vi "LabVIEW Basics #1 - Arduino Blinking LED.vi"() -> ()   [LabVIEW 2019]
uses:
  <vilib>/MakerHub/LINX/Public/Peripherals/Digital/Digital Write 1 Chan.vi
  <vilib>/MakerHub/LINX/Public/Peripherals/Digital/Digital Write N Chans.vi
  <vilib>/MakerHub/LINX/Private/Local IO/LinxDigitalWrite.vi
  <vilib>/MakerHub/LINX/Public/Utilities/Check Channel.vi
  <vilib>/MakerHub/LINX/Public/Utilities/Open Serial.vi
  <vilib>/MakerHub/LINX/Private/Utilties/Generate Error.vi
  <vilib>/MakerHub/LINX/LMH-LINX.lvlib
panel:
  in  "Frequency (Hz)":dbl(slide)=1.0 min=1.0 max=10.0 step=1.0 scale=1.0..10.0
  out "LED":bool
  out "Device Name":string
  in  "Stop":bool
  # "Indicators"
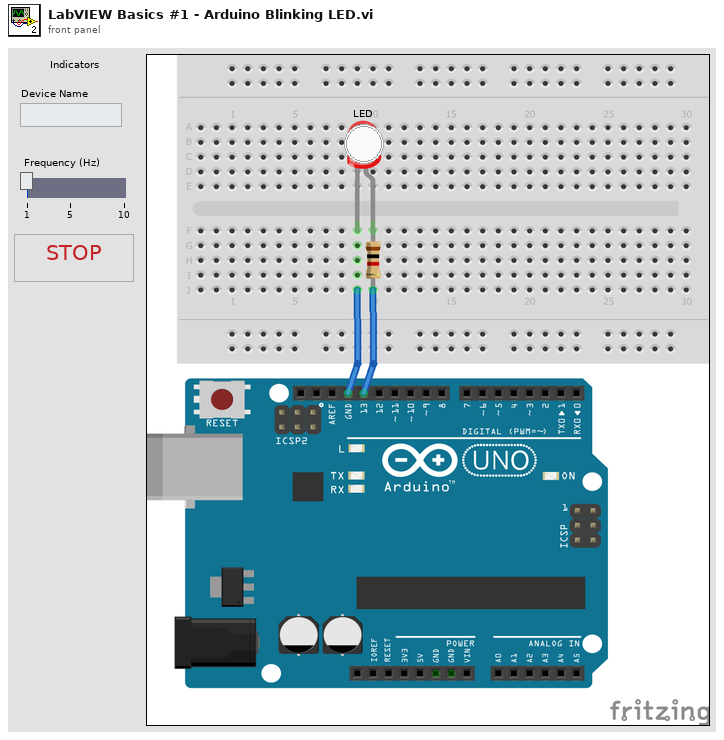
[diagram p1: front panel]
types:
  T1 = typedef "LMH-LINX.lvlib/LINX Ref.ctl" = cluster{"IO":T2, "Interface":T3, "LINX Device Config":T4}
  T2 = typedef "LMH-LINX.lvlib/Platform.ctl" = enum16{"Remote", "Local"}
  T3 = typedef "LMH-LINX.lvlib/Interface.ctl" = enum16{"Serial", "TCP"}
  T4 = typedef "LMH-LINX.lvlib/Device.lvlib/LINX Device Config.ctl" = cluster{"Interface":T3, "COM Port":refnum<visa-resource-name>, "TCP Configuration":T5, "Device Family":u8, "Device ID":u8, "Device Name":string, "TCP Ref":refnum<k5>, "Channels":T6}
  T5 = typedef "LMH-LINX.lvlib/Device.lvlib/TCP Config.ctl" = cluster{"IP Address":string, "Port":u16}
  T6 = typedef "LMH-LINX.lvlib/Channels.ctl" = cluster{"DI":u8[], "DO":u8[], "AI":u8[], "AO":u8[], "PWM":u8[], "QE":u8[], "UART":u8[], "I2C 2":u8[], "SPI":u8[], "CAN":u8[], "Servo":u8[], "AI Ref (V)":dbl, "AI Resolution (Bits)":u8, "AO Ref (V)":dbl, "AO Resolution (Bits)":u8}
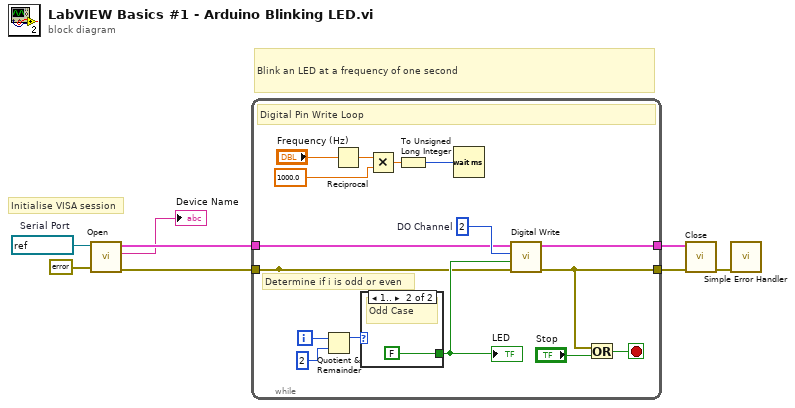
[diagram p0: block diagram]
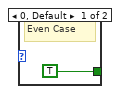
[diagram p2: hidden frame]
diagram:
  w6 = refnum<visa-resource-name> "COM6"  # Serial Port
  # "Initialise VISA session"
  # "Blink an LED at a frequency of one second"
  n1 = call-poly <vilib>:"Open.vi"("Error In"=errorcluster {"status"=FALSE, "code"=0, "source"=""}, "Serial Port"=w6) -> ("Error Out"=w7:errorcluster, "Device Name"=→"Device Name":string, "LINX Resource"=w8:T1)  [unwired: 7 in]
  n2 = while {
    tunnel: w8 -> [w12]
    tunnel: [w11] -> _
    tunnel: w7 -> [w11]
    tunnel: [w21] -> w5
    tunnel: [w22] -> w4
    i -> [w10]
    stop <- w23 stop-if-true
    w20 = u8 2  # DO Channel
    # "Determine if i is odd or even"
    # "Digital Pin Write Loop"
    n3 = Quotient & Remainder(x=w10, y=2) -> (x-y*floor(x/y)=w18:i32)  [unwired: 1 out]
    n4 = Reciprocal(x="Frequency (Hz)") -> (1/x=w16:dbl)
    n5 = case shown="1.." w18 {
      tunnel: [TRUE FALSE] -> w17
      frame 0, Default {
        # "Even Case"
      }
      frame 1.. {
        # "Odd Case"
      }
    }
    "LED" <- w17
    n6 = Multiply(x=w16, y=1000.0) -> (x*y=w13:dbl)
    n7 = To Unsigned Long Integer(number=w13) -> (unsigned 32bit integer=w9:u32)
    n8 = Wait (ms)(milliseconds to wait=w9) -> ()  [unwired: 1 out]
    n9 = call-poly <vilib>:"Digital Write.vi"("Error In"=w11, "Output Value"=w17, "DO Channel"=w20, "LINX Resource"=w12) -> ("Error Out"=w22:errorcluster, "LINX Resource"=w21:T1)  [unwired: 6 in]
    n10 = Or(x=w22, y="Stop") -> (x .or. y?=w23:bool)
  }
  n11 = call <vilib>:"Close.vi"("Error In"=w4, "LINX Resource"=w5) -> ("Error Out"=w1:errorcluster)  [unwired: 9 in]
  n12 = call <vilib>:"Simple Error Handler.vi"("error in (no error)"=w1) -> ()  [unwired: 4 in, 5 out]
